vi "Status Update.vi"(1 "Exp Status":T2 {"Saving" items=["N.A.", "OK", "Busy", "Done"]; "Plotting" items=["N.A.", "OK", "Busy", "Done"]; "Buffer" items=["N.A.", "OK", "Busy", "Done"]; "Exposure" items=["N.A.", "OK", "Busy", "Done"]; "Spectrometer" items=["N.A.", "OK", "Busy", "Done"]; "Temperature" items=["N.A.", "OK", "Busy", "Done"]; "Field" items=["N.A.", "OK", "Busy", "Done"]}) -> (0 "Exp Status output":T2 {"Saving" items=["N.A.", "OK", "Busy", "Done"]; "Plotting" items=["N.A.", "OK", "Busy", "Done"]; "Buffer" items=["N.A.", "OK", "Busy", "Done"]; "Exposure" items=["N.A.", "OK", "Busy", "Done"]; "Spectrometer" items=["N.A.", "OK", "Busy", "Done"]; "Temperature" items=["N.A.", "OK", "Busy", "Done"]; "Field" items=["N.A.", "OK", "Busy", "Done"]})   [LabVIEW 2020]
uses:
  Globals and TypeDefs/Type Definitions.llb/3 way Status.ctl
  Globals and TypeDefs/gStatus.vi
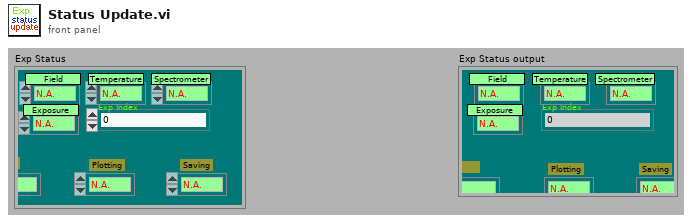
[diagram p1: front panel]
types:
  T1 = typedef "3 way Status.ctl" = u8
  T2 = cluster{"Exp Index":u32, "Field":T1, "Temperature":T1, "Spectrometer":T1, "Exposure":T1, "Buffer":T1, "Plotting":T1, "Saving":T1}
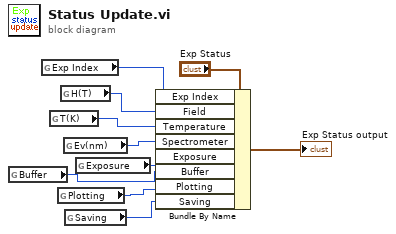
[diagram p0: block diagram]
diagram:
  n1 = global read "gStatus.vi" "Buffer"() -> (w5:T1)
  n2 = global read "gStatus.vi" "Exp Index"() -> (w2:u32)
  n3 = global read "gStatus.vi" "T(K)"() -> (w8:T1)
  n4 = global read "gStatus.vi" "Plotting"() -> (w4:T1)
  n5 = global read "gStatus.vi" "H(T)"() -> (w3:T1)
  n6 = global read "gStatus.vi" "Ev(nm)"() -> (w7:T1)
  n7 = global read "gStatus.vi" "Saving"() -> (w1:T1)
  n8 = global read "gStatus.vi" "Exposure"() -> (w6:T1)
  n9 = Bundle By Name(cluster="Exp Status", "Exp Index"=w2, "Field"=w3, "Temperature"=w8, "Spectrometer"=w7, "Exposure"=w6, "Buffer"=w5, "Plotting"=w4, "Saving"=w1) -> (→"Exp Status output":T2)
